vi "Player Info.vi"(11 "Galaxy in":refnum<class "Galaxy.lvclass">) -> (0 "Defeat Speech":string, 1 "Victory Speech":string, 2 "Name":string, 3 "Galaxy out":refnum<class "Galaxy.lvclass">)   [LabVIEW 2020, in "Galaxy.lvclass"]
uses:
  Galaxy.lvclass
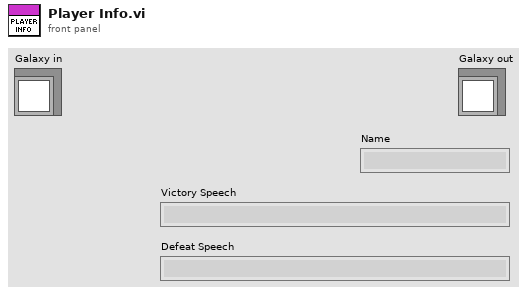
[diagram p1: front panel]
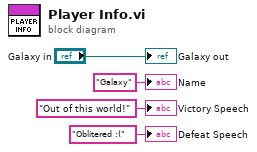
[diagram p0: block diagram]
diagram:
  "Galaxy out" <- "Galaxy in"
  "Name" <- "Galaxy" ("Name")
  "Victory Speech" <- "Out of this world!" ("Victory Speech")
  "Defeat Speech" <- "Oblitered :(" ("Defeat Speech")
